vi "Read_Helium gas meter remotely.vi"() -> ()   [LabVIEW 2015]
uses:
  <vilib>/Platform/TimedLoop/XDataNode/timing_clust.ctl
  <vilib>/Platform/TimedLoop/XDataNode/nitl_modes.ctl
  <vilib>/Platform/TimedLoop/XDataNode/wakeup.ctl
  <vilib>/Utility/file.llb/Write To Spreadsheet File (DBL).vi
  <vilib>/Utility/file.llb/Read From Spreadsheet File (DBL).vi
  <vilib>/platform/TimedLoop/XDataNode/XDataNode.xnode
  <vilib>/Platform/TimedLoop/XDataNode/XDNodeRunTimeDep.lvlib
panel:
  in  "Graph on/off":bool
  in  "URL 2":string="http://130.55.69.25"
  out "CuFt Ghz Lab":dbl
  in  "file path (dialog if empty)":path=path "C:/Data/Bag gas meter.dat"
  out "XY Graph":cluster{"all rows":dbl[], "all rows":dbl[]}[](graph)
  out "CuFt Bag":dbl
  in  "URL":string="http://130.55.69.22"
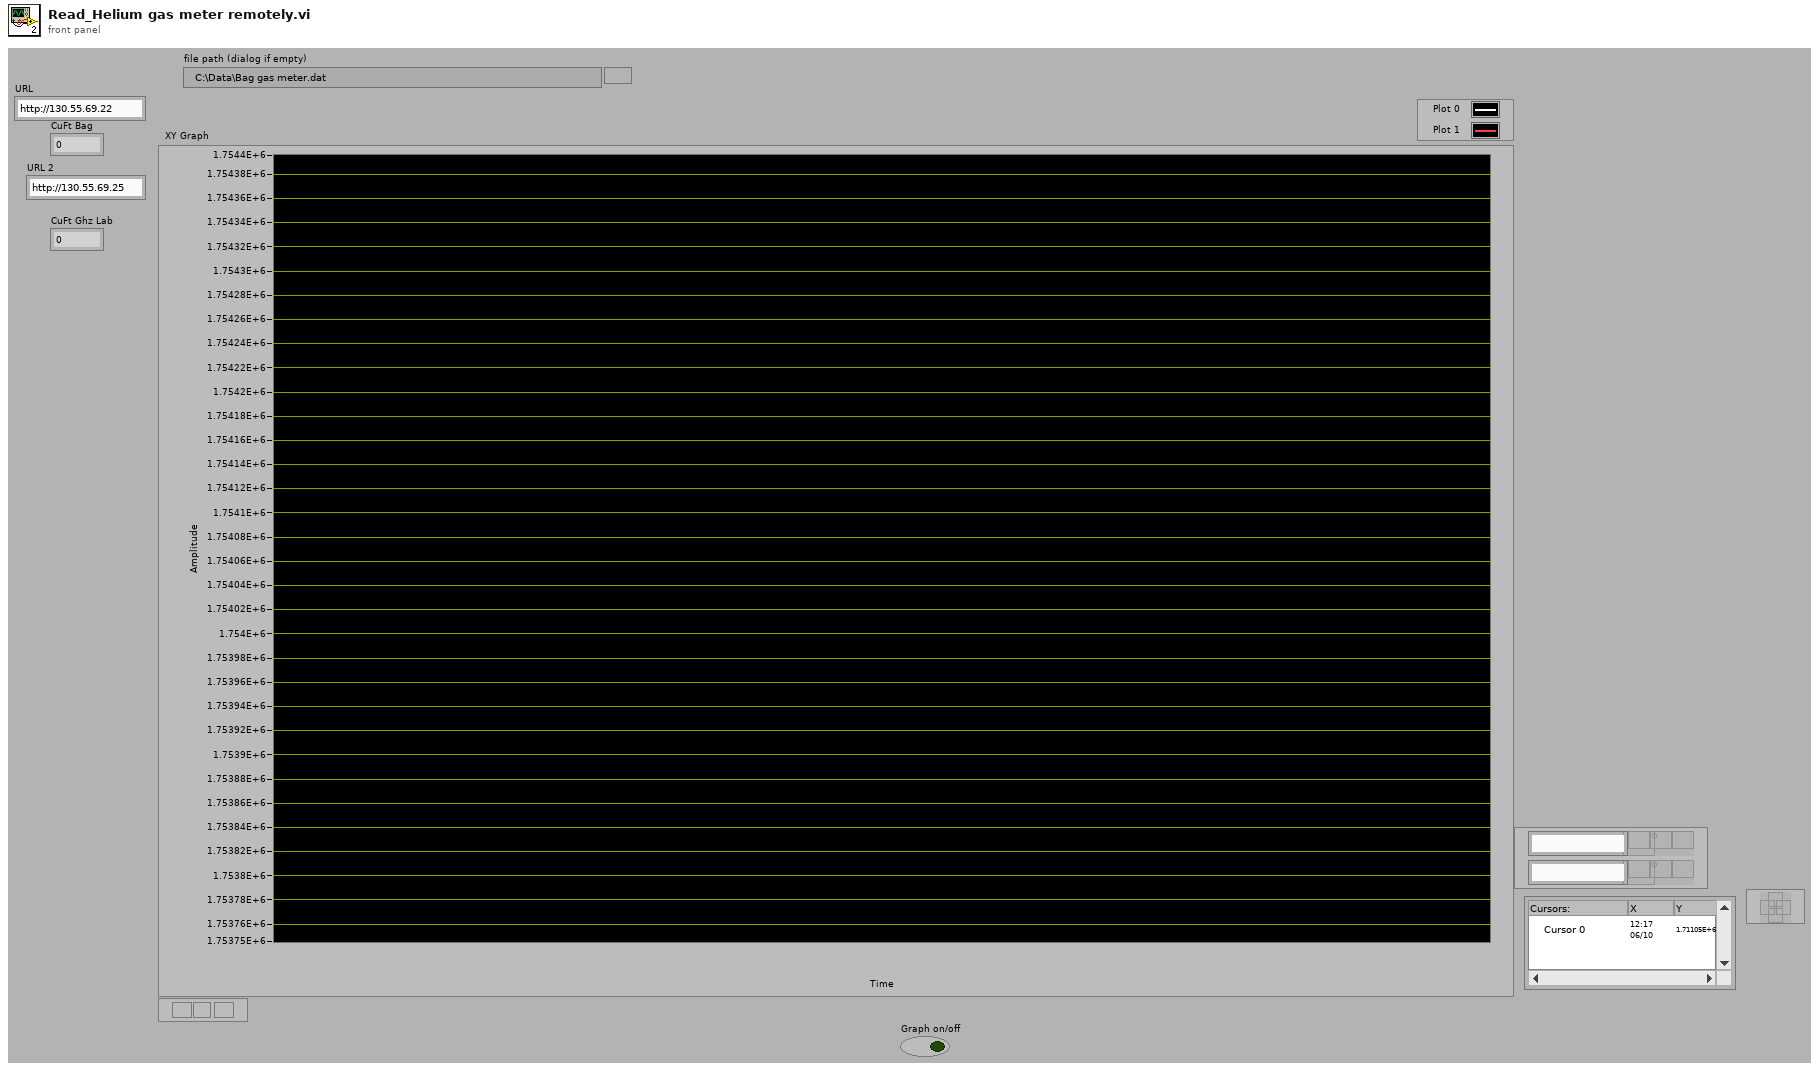
[diagram p1: front panel]
types:
  T1 = typedef "XDNodeRunTimeDep.lvlib/timing_clust.ctl" = cluster{"Expected End [f-1]":u64, "Actual End [f-1]":u64, "Finished Late? [f-1]":bool, "Expected End [i-1]":u64, "Actual End [i-1]":u64, "Finished Late? [i-1]":bool, "Expected Start [i]":u64, "Actual Start [i]":u64, "Expected Start [f]":u64, "Actual Start [f]":u64, "Source Name":string, "Structure Name":string, "Period":i64, "Deadline":i64, "Offset":i64, "Start":i64, "Priority":i32, "Timeout":i32, "Mode":T2, "Wakeup Reason":T3, "Error":errorcluster, "Source Type":string, "Secondary Source Type":string, "Global End Time":u64, "Global Start Time":u64, "Frame Duration":u64, "Iteration Duration":u64, "Assigned CPU":i32, "I/O Scan Engine Mode":u32}
  T2 = typedef "XDNodeRunTimeDep.lvlib/nitl_modes.ctl" = enum32{"No Change", "Process missed periods, maintain original phase", "Discard missed periods, maintain original phase", "Process missed periods, ignore original phase", "Discard missed periods, ignore original phase"}
  T3 = typedef "XDNodeRunTimeDep.lvlib/wakeup.ctl" = enum32{"Normal", "Aborted", "Asynchronous wakeup", "Timing source error", "Timed loop error", "Timeout"}
  T4 = enum16{"Read", "Write", "ReadWrite", "BufferedRead", "BufferedReadWrite"}
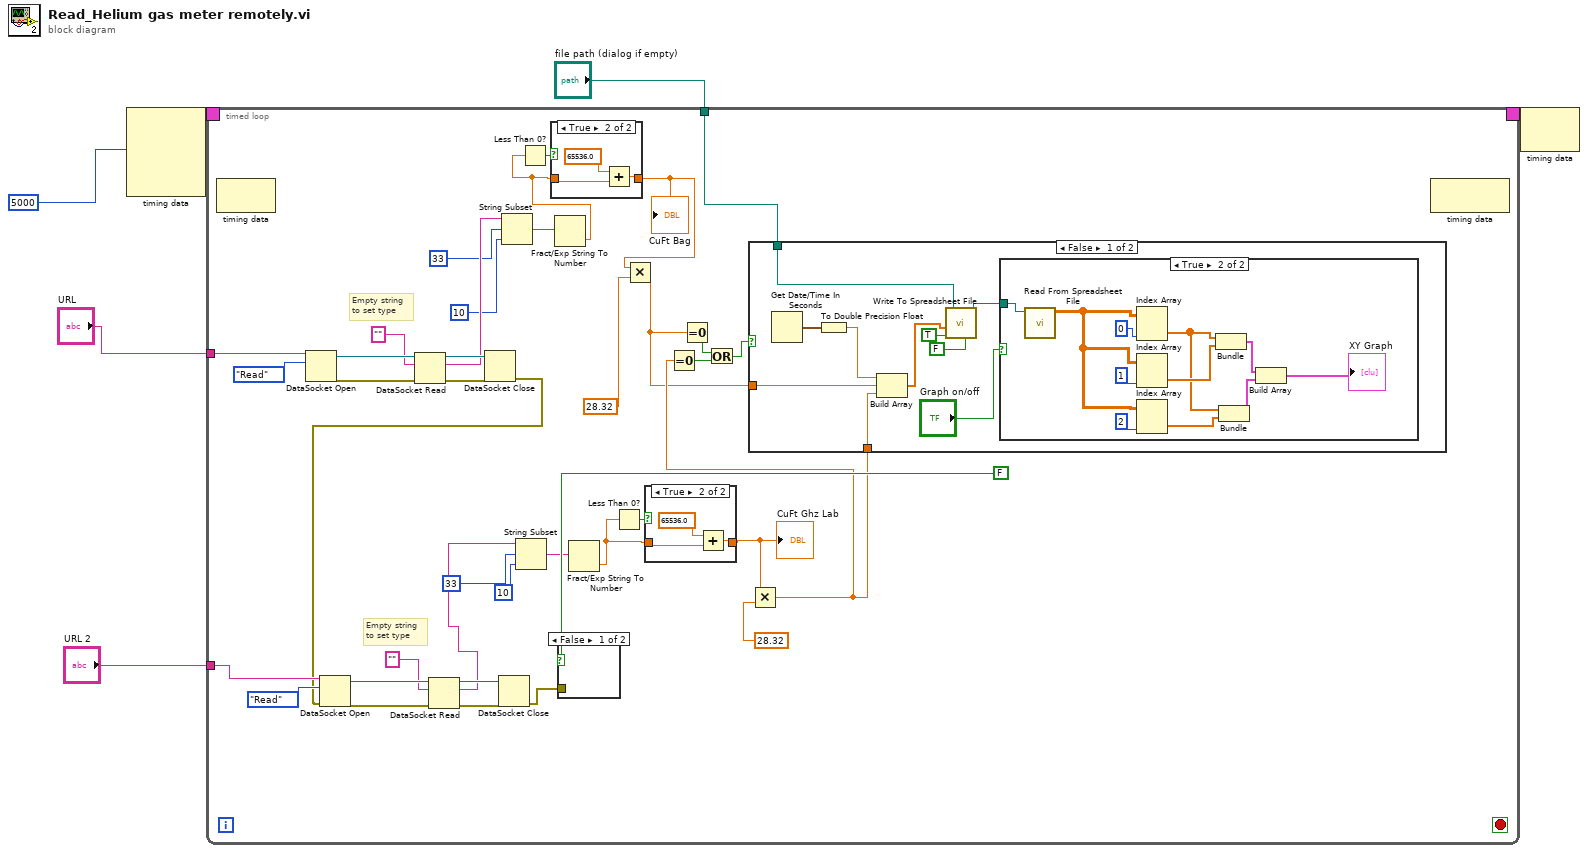
[diagram p0: block diagram]
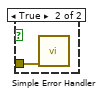
[diagram p6: hidden frame]
diagram:
  n1 = node-c288(i64 5000 ("Period")) -> (w5:T1)  [unwired: 3 in]
  n2 = timed-loop {
    timing: w5 -> [_]
    timing-out: [_] -> w4
    tunnel: "URL" -> [w39]
    tunnel: "file path (dialog if empty)" -> [w33]
    tunnel: "URL 2" -> [w20]
    stop <- _ stop-if-true
    # "Empty string\nto set type"
    # "Empty string\nto set type"
    n3 = node-c288() -> ()  [unwired: 1 in, 1 out]
    n4 = DataSocket Open(10:T4."Read" ("mode"), 11:w39) -> (0:w42:errorcluster, 3:w45:refnum<k13>)  [unwired: 2 in]
    n5 = DataSocket Read(8:w42, 10:"", 11:w45) -> (0:w43:errorcluster, 2:w38:string, 3:w44:refnum<k13>)  [unwired: 2 in, 4 out]
    n6 = DataSocket Close(8:w43, 11:w44) -> (0:w19:errorcluster)  [unwired: 1 in, 1 out]
    n7 = DataSocket Open(8:w19, 10:T4."Read" ("mode"), 11:w20) -> (0:w28:errorcluster, 3:w31:refnum<k13>)  [unwired: 1 in]
    n8 = DataSocket Read(8:w28, 10:"", 11:w31) -> (0:w29:errorcluster, 2:w25:string, 3:w30:refnum<k13>)  [unwired: 2 in, 4 out]
    n9 = DataSocket Close(8:w29, 11:w30) -> (0:w18:errorcluster)  [unwired: 1 in, 1 out]
    n10 = String Subset(string=w38, offset (0)=33, length (rest)=10 ("length (rest)")) -> (substring=w35:string)
    n11 = String Subset(string=w25, offset (0)=33 ("offset (0) 2"), length (rest)=10 ("length (rest) 2")) -> (substring=w22:string)
    n12 = Fract/Exp String To Number(string=w35) -> (number=w8:dbl)  [unwired: 3 in, 1 out]
    n13 = Less Than 0?(x=w8) -> (x < 0?=w9:bool)
    n14 = case shown="True" w9 {
      tunnel: w8 -> [w46 w48]
      tunnel: [w46 w49] -> w7
      frame False {
      }
      frame True {
        n15 = Add(x=65536.0, y=w48) -> (x+y=w49:dbl)
      }
    }
    "CuFt Bag" <- w7
    n16 = case shown="False" FALSE {
      tunnel: w18 -> [_ w75]
      frame False {
      }
      frame True {
        n17 = call <vilib>:"Simple Error Handler.vi"("error in (no error)"=w75) -> ()  [unwired: 4 in, 5 out]
      }
    }
    n18 = Fract/Exp String To Number(string=w22) -> (number=w11:dbl)  [unwired: 3 in, 1 out]
    n19 = Less Than 0?(x=w11) -> (x < 0?=w12:bool)
    n20 = Multiply(x=w7, y=28.32) -> (x*y=w14:dbl)
    n21 = case shown="True" w12 {
      tunnel: w11 -> [w50 w52]
      tunnel: [w50 w53] -> w10
      frame False {
      }
      frame True {
        n22 = Add(x=65536.0, y=w52) -> (x+y=w53:dbl)
      }
    }
    "CuFt Ghz Lab" <- w10
    n23 = Equal To 0?(x=w14) -> (x = 0?=w17:bool)
    n24 = Multiply(x=w10, y=28.32) -> (x*y=w15:dbl)
    n25 = Equal To 0?(x=w15) -> (x = 0?=w16:bool)
    n26 = Or(x=w17, y=w16) -> (x .or. y?=w13:bool)
    n27 = case shown="False" w13 {
      tunnel: w33 -> [w62 _]
      tunnel: w14 -> [w57 _]
      tunnel: w15 -> [w55 _]
      frame False {
        n28 = Get Date/Time In Seconds() -> (seconds since 1Jan1904=w63:timestamp)
        n29 = To Double Precision Float(number=w63) -> (double precision float=w56:dbl)
        n30 = Build Array(w56, w57, w55) -> (w59:dbl[])
        n31 = call-poly <vilib>:"Write To Spreadsheet File.vi"("transpose? (no:F)"=FALSE, "append to file? (new file:F)"=TRUE, "1D data"=w59, "file path (dialog if empty)"=w62) -> ("new file path (Not A Path if cancelled)"=w58:path)  [unwired: 4 in]
        n32 = case shown="True" "Graph on/off" {
          tunnel: w58 -> [_ w74]
          frame False {
          }
          frame True {
            n33 = call-poly <vilib>:"Read From Spreadsheet File.vi"("file path (dialog if empty)"=w74) -> ("all rows"=w68:dbl[][])  [unwired: 6 in, 4 out]
            n34 = Index Array(array=w68, index (col)=0 ("index (row)")) -> (element=w67:dbl[])  [unwired: 1 in]
            n35 = Index Array(array=w68, index (col)=1 ("index (row)")) -> (element=w73:dbl[])  [unwired: 1 in]
            n36 = Index Array(array=w68, index (col)=2 ("index (row)")) -> (element=w69:dbl[])  [unwired: 1 in]
            n37 = Bundle("all rows"=w67, "all rows"=w73) -> (w66:cluster{"all rows":dbl[], "all rows":dbl[]})  [unwired: 1 in]
            n38 = Bundle("all rows"=w67, "all rows"=w69) -> (w65:cluster{"all rows":dbl[], "all rows":dbl[]})  [unwired: 1 in]
            n39 = Build Array(w66, w65) -> (→"XY Graph":cluster{"all rows":dbl[], "all rows":dbl[]}[])
          }
        }
      }
      frame True {
      }
    }
    n40 = node-c288() -> ()  [unwired: 1 in, 1 out]
  }
  n41 = node-c288(w4) -> ()  [unwired: 1 out]
